vi "PWM Out.vi"() -> ()   [LabVIEW 2016]
doc: "This VI generates a pulse width modulated output with variable high and low periods. The potentiometer is used to vary the duty cycle from 0% to 100%. The first toggle switch is used to switch between .5 Hz and 100 Hz PWM frequencies.\n\nThe output will be shown on the eight LEDs of the sbRIO evaluation board."
uses:
  <vilib>/rvi/Emulation/niFpgaGetClockAttributes.vi
  <vilib>/rvi/Emulation/niFpgaSctlEmulationGetInTimedLoop.vi
  <vilib>/rvi/Emulation/niFpgaEmulationReportErrorSimple.vi
  <vilib>/rvi/eio/common/nirviEmuTemplateMethod_errors.vi
  <vilib>/rvi/Emulation/niFpgaCriticalErrorInLSC.vi
  <vilib>/eio/EIONode/EIONode.xnode
panel:
  out "Duty Cycle":fxp<+/-,64,12> format="%.56g"
  out "Period (us)":u32
  out "High Period (us)":u32
  out "Low Period (us)":u32
  # "This VI generates a pulse width modulated output with variable high\nand low periods.  The potentiometer is used to vary the duty cycle \nfrom 0% to 100% (0-1). Keep the Duty Cycle below 1 for normal \nexecution. The first toggle switch is used to switch between .5 Hz \nand 100 Hz PWM frequencies.\n\nThe output will be shown on the eight LEDs of the LabVIEW RIO \nevaluation board."
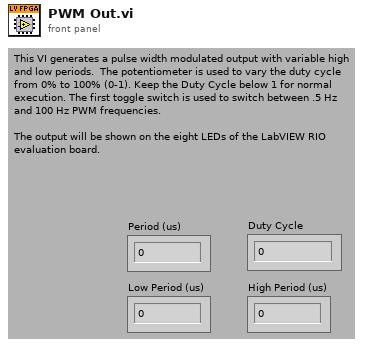
[diagram p1: front panel]
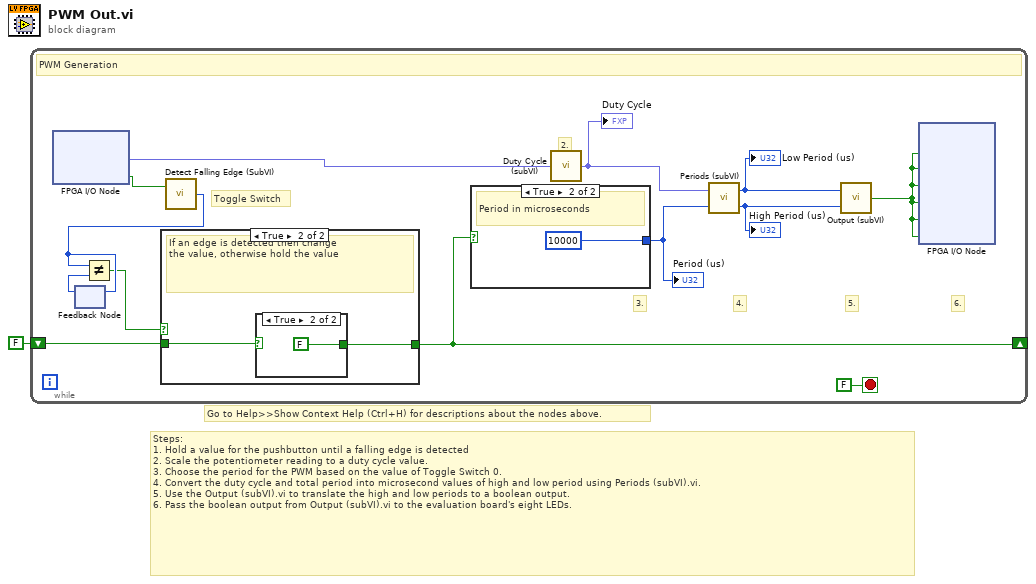
[diagram p0: block diagram]
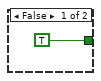
[diagram p3: hidden frame]
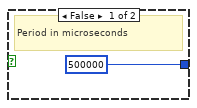
[diagram p4: hidden frame]
diagram:
  # "Go to Help>>Show Context Help (Ctrl+H) for descriptions about the nodes above."
  # "Steps:\n1. Hold a value for the pushbutton until a falling edge is detected\n2. Scale the potentiometer reading to a duty cycle value.\n3. Choose the period for the PWM based on the value of Toggle Switch 0.\n4. Convert the duty cycle and total period into microsecond values of high and low period using Periods (subVI).vi.\n5. Use the Output (subVI).vi to translate the high and low periods to a boolean output.\n6. Pass the boolean output from Output (subVI).vi to the evaluation board's eight LEDs."
  n1 = while {
    shift-right: [w2] -> _
    shift-left: FALSE -> [w7]
    stop <- FALSE ("stop") stop-if-true
    # "6."
    # "5."
    # "Toggle Switch"
    # "4."
    # "3."
    # "2."
    # "PWM Generation"
    n2 = xnode "FPGA I/O Node"() -> ("POT"=w8:fxp<+/-,24,5>, "PB1"=w3:bool)  [unwired: 2 in, 2 out]
    n3 = feedback #1() -> (w5:u8)  [unwired: 1 in]
    n4 = call "Detect Falling Edge (SubVI).vi"("Trigger"=w3) -> ("8-bit Count (0-63)"=w6:u8)  [unwired: 1 in]
    n5 = feedback-in #1(w6) -> ()
    n6 = Not Equal?(x=w6, y=w5) -> (x != y?=w4:bool)
    n7 = case shown="True" w4 {
      tunnel: w7 -> [w15 w17]
      tunnel: [w15 w16] -> w2
      frame False {
        # "hold the value"
      }
      frame True {
        # "If an edge is detected then change \nthe value, otherwise hold the value"
        n8 = case shown="True" w17 {
          tunnel: [TRUE FALSE] -> w16
          frame False {
          }
          frame True {
          }
        }
      }
    }
    n9 = case shown="True" w2 {
      tunnel: [u32 500000 u32 10000] -> w12
      frame False {
        # "Period in microseconds"
      }
      frame True {
        # "Period in microseconds"
      }
    }
    "Period (us)" <- w12
    n10 = call "Duty Cycle (subVI).vi"("Potentiometer"=w8) -> ("Duty Cycle"=w13:fxp<+/-,64,12>)
    "Duty Cycle" <- w13
    n11 = call "Periods (subVI).vi"("Period (usec)"=w12, "Duty Cycle"=w13) -> ("High Period (us)"=w10:u32, "Low Period (us)"=w11:u32)
    "Low Period (us)" <- w11
    "High Period (us)" <- w10
    n12 = call "Output (subVI).vi"("High Period (us)"=w10, "Low Period (us)"=w11) -> ("Output 0"=w9:bool)
    n13 = xnode "FPGA I/O Node"("LED 1"=w9, "LED 2"=w9, "LED 3"=w9, "LED 4"=w9, "LED 5"=w9, "LED 6"=w9) -> ()  [unwired: 6 in, 6 out]
  }
